vi "fstat.vi"(8 "error in (no error)":errorcluster, 11 "file descriptor":i32) -> (0 "error out":errorcluster, 3 "stat":T1)   [LabVIEW 2013, in "Linux RT IPC.C.lvlib"]
doc: "Wrapper VI for Linux function fstat()."
uses:
  Linux RT IPC.C.lvlib
  Controls/C Types/stat_64.ctl
  Controls/C Types/dev_t.ctl
  Controls/C Types/ino_t_64.ctl
  Controls/C Types/mode_t.ctl
  Controls/C Types/nlink_t_64.ctl
  Controls/C Types/uid_t.ctl
  Controls/C Types/gid_t.ctl
  Controls/C Types/off_t_64.ctl
  Controls/C Types/blksize_t_64.ctl
  Controls/C Types/blkcnt_t_64.ctl
  Controls/C Types/time_t_64.ctl
  Controls/C Types/stat_32.ctl
  Controls/C Types/ino_t_32.ctl
  Controls/C Types/nlink_t_32.ctl
  Controls/C Types/off_t_32.ctl
  Controls/C Types/blksize_t_32.ctl
  Controls/C Types/blkcnt_t_32.ctl
  Controls/C Types/time_t_32.ctl
  Controls/functions.ctl
  <vilib>/NI/NI Linux RT Errno/Linux Errno.lvlib
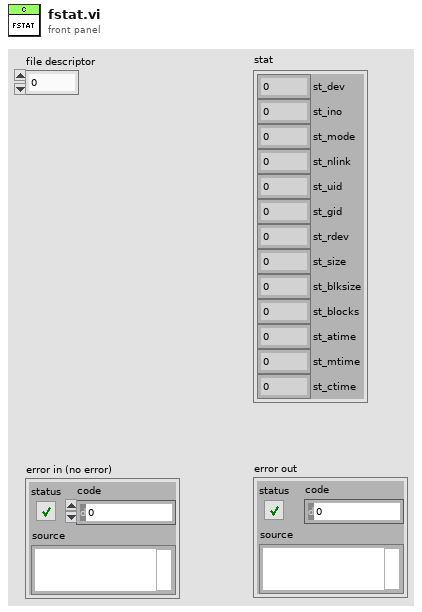
[diagram p1: front panel]
types:
  T1 = typedef "Linux RT IPC.C.lvlib/stat_64.ctl" = cluster{"st_dev":T2, "st_ino":T3, "st_mode":T4, "st_nlink":T5, "st_uid":T6, "st_gid":T7, "st_rdev":T2, "st_size":T8, "st_blksize":T9, "st_blocks":T10, "st_atime":T11, "st_mtime":T11, "st_ctime":T11}
  T2 = typedef "Linux RT IPC.C.lvlib/dev_t.ctl" = u64
  T3 = typedef "Linux RT IPC.C.lvlib/ino_t_64.ctl" = u64
  T4 = typedef "Linux RT IPC.C.lvlib/mode_t.ctl" = u32
  T5 = typedef "Linux RT IPC.C.lvlib/nlink_t_64.ctl" = u64
  T6 = typedef "Linux RT IPC.C.lvlib/uid_t.ctl" = u32
  T7 = typedef "Linux RT IPC.C.lvlib/gid_t.ctl" = u32
  T8 = typedef "Linux RT IPC.C.lvlib/off_t_64.ctl" = u64
  T9 = typedef "Linux RT IPC.C.lvlib/blksize_t_64.ctl" = u64
  T10 = typedef "Linux RT IPC.C.lvlib/blkcnt_t_64.ctl" = u64
  T11 = typedef "Linux RT IPC.C.lvlib/time_t_64.ctl" = u64
  T12 = typedef "Linux RT IPC.C.lvlib/stat_32.ctl" = cluster{"st_dev":T2, "st_ino":T13, "st_mode":T4, "st_nlink":T14, "st_uid":T6, "st_gid":T7, "st_rdev":T2, "st_size":T15, "st_blksize":T16, "st_blocks":T17, "st_atime":T18, "st_mtime":T18, "st_ctime":T18}
  T13 = typedef "Linux RT IPC.C.lvlib/ino_t_32.ctl" = u32
  T14 = typedef "Linux RT IPC.C.lvlib/nlink_t_32.ctl" = u32
  T15 = typedef "Linux RT IPC.C.lvlib/off_t_32.ctl" = u32
  T16 = typedef "Linux RT IPC.C.lvlib/blksize_t_32.ctl" = u32
  T17 = typedef "Linux RT IPC.C.lvlib/blkcnt_t_32.ctl" = u32
  T18 = typedef "Linux RT IPC.C.lvlib/time_t_32.ctl" = u32
  T19 = typedef "Linux RT IPC.C.lvlib/functions.ctl" = enum16{"unspecified", "close", "epoll_create", "epoll_ctl", "epoll_wait", "fstat", "ftruncate", "mkfifo", "mmap", "munmap", "open", "read", "shm_open", "shm_unlink", "timerfd_create", "timerfd_settime", "timerfd_gettime", "write", "unlink"}
  T20 = typedef "Linux Errno.lvlib/errno.ctl" = enum16{"NO ERROR", "EPERM", "ENOENT", "ESRCH", "EINTR", "EIO", "ENXIO", "E2BIG", "ENOEXEC", "EBADF", "ECHILD", "EAGAIN", "ENOMEM", "EACCES", "EFAULT", "ENOTBLK", "EBUSY", "EEXIST", "EXDEV", "ENODEV", "ENOTDIR", "EISDIR", "EINVAL", "ENFILE", "EMFILE", "ENOTTY", "ETXTBSY", "EFBIG", "ENOSPC", "ESPIPE", "EROFS", "EMLINK", "EPIPE", "EDOM", "ERANGE", "EDADLK", "ENAMETOOLONG", "ENOLCK", "ENOSYS", "ENOTEMPTY", "ELOOP", "EWOULDBLOCK", "ENOMSG", "EIDRM", "ECHRNG", "EL2NSYNC", "EL3HLT", "EL3RST", "ELNRNG", "EUNATCH", "ENOCSI", "EL2HLT", "EBADE", "EBADR", "EXFULL", "ENOANO", "EBADRQC", "EBADSLT", "EDEADLOCK", "EBFONT", "ENOSTR", "ENODATA", "ETIME", "ENOSR", "ENONET", "ENOPKG", "EREMOTE", "ENOLINK", "EADV", "ESRMNT", "ECOMM", "EPROTO", "EMULTIHOP", "EDOTDOT", "EBADMSG", "EOVERFLOW", "ENOTUNIQ", "EBADFD", "EREMCHG", "ELIBACC", "ELIBBAD", "ELIBSCN", "ELIBMAX", "ELIBEXEC", "ELISEQ", "ERESTART", "ESTRPIPE", "EUSERS", "ENOTSOCK", "EDESTADDRREQ", "EMSGSIZE", "EPROTOTYPE", "ENOPROTOOPT", "EPROTONOSUPPORT", "ESOCKTNOSUPPORT", "EOPNOTSUPP", "EPFNOSUPPORT", "EAFNOSUPPORT", "EADDRINUSE", "EADDRNOTAVAIL", "ENETDOWN", "ENETUNREACH", "ENETRESET", "ECONNABORTED", "ECONNRESET", "ENOBUFS", "EISCONN", "ENOTCONN", "ESHUTDOWN", "ETOOMANYREFS", "ETIMEDOUT", "ECONNREFUSED", "EHOSTDOWN", "EHOSTUNREACH", "EALREADY", "EINPROGRESS", "ESTALE", "EUCLEAN", "ENOTNAM", "ENAVAIL", "EISNAM", "EREMOTEIO", "EDQUOT", "ENOMEDIUM", "EMEDIUMTYPE", "ECANCELED", "ENOKEY", "EKEYEXPIRED", "EKEYREVOKED", "EKEYREJECTED", "EOWNERDEAD", "ENOTRECOVERABLE", "ERFKILL", "EHWPOISON", "UNDEFINED"}
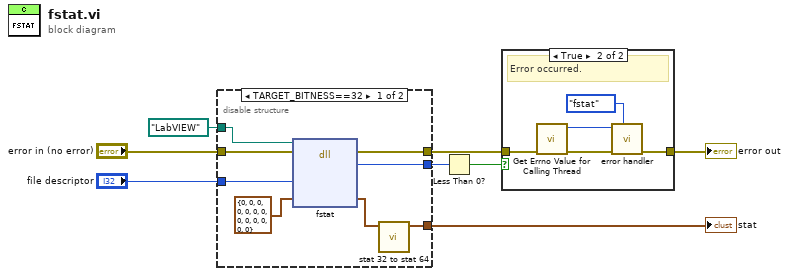
[diagram p0: block diagram]
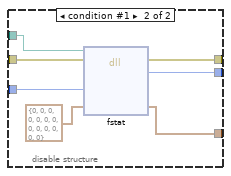
[diagram p3: hidden frame]
diagram:
  n1 = disable-structure shown="TARGET_BITNESS==32" {
    disable-tunnel: "error in (no error)" -> [w16 w23]
    disable-tunnel: "file descriptor" -> [w15 w22]
    disable-tunnel: path "LabVIEW" ("path to libc") -> [w9 w21]
    disable-tunnel: [w12 w19] -> w5
    disable-tunnel: [w11 w17] -> w3
    disable-tunnel: [w10 w18] -> w4
    frame condition #0 (active) {
      n2 = dll-call lib="?" fn="fstat"(path in=w9, error in=w16, "fd"=w15, "stat"=T12 {"st_dev"=0, "st_ino"=0, "st_mode"=0, "st_nlink"=0, "st_uid"=0, "st_gid"=0, "st_rdev"=0, "st_size"=0, "st_blksize"=0, "st_blocks"=0, "st_atime"=0, "st_mtime"=0, "st_ctime"=0}) -> (error out=w11:errorcluster, "status"=w10:i32, "stat"=w13:T12)  [unwired: 2 in, 1 out]
      n3 = call "stat 32 to stat 64.vi"("stat 32"=w13) -> ("stat 64"=w12:T1)  [unwired: 10 in]
    }
    frame condition #1 {
      n4 = dll-call lib="?" fn="fstat"(path in=w21, error in=w23, "fd"=w22, "stat"=T1 {"st_dev"=0, "st_ino"=0, "st_mode"=0, "st_nlink"=0, "st_uid"=0, "st_gid"=0, "st_rdev"=0, "st_size"=0, "st_blksize"=0, "st_blocks"=0, "st_atime"=0, "st_mtime"=0, "st_ctime"=0} ("stat 2")) -> (error out=w17:errorcluster, "status"=w18:i32, "stat"=w19:T1)  [unwired: 2 in, 1 out]
    }
  }
  "stat" <- w5
  n5 = Less Than 0?(x=w4) -> (x < 0?=w2:bool)
  n6 = case shown="True" w2 {
    tunnel: w3 -> [w24 w29]
    tunnel: [w24 w27] -> w7
    frame False {
      # "No error."
    }
    frame True {
      # "Error occurred."
      n7 = call <vilib>:"Get Errno Value for Calling Thread.vi"("error in (no error)"=w29) -> ("error out"=w28:errorcluster, "errno"=w26:T20)  [unwired: 9 in]
      n8 = call "error handler.vi"("function (unspecified)"=functions."fstat", "error in (no error)"=w28, "errno"=w26) -> ("error out"=w27:errorcluster)  [unwired: 8 in]
    }
  }
  "error out" <- w7
